vi "__package_structure.vi"(1 "data":string="Single shunt, R(Z1), 1kohm, S/N: 5\u0000\u0000                                                                                                                                                                                                                                                                                                                                                                                                                                                                                                                                                                                                                                                                                                                                                                                                                                                                                                                                                                                                    í\u0004\u0001\u0001\u0001\u0000\u0000\u0000\u0000\u0000\u0000?\u0007zD²ôç´\u0000\u0000?\u0007zD²ôgµ\u0000\u0000\u0000@\u0007zD²ôçµ\u0000\u0000@\u0007zD²ôg¶\u0000\u0000\u0000A\u0007zD²ôç¶\u0000\u0000A\u0007zD²ôg·\u0000\u0000\u0000B\u0007zD²ôç·\u0000\u0000B\u0007zD²ôg¸\u0000\u0000\u0000C\u0007zD²ôç¸\u0000\u0000C\u0007zD²ôg¹\u0000\u0000\u0000D\u0007zD²ôç¹\u0000\u0000D\u0007zD²ôgº\u0000\u0000\u0000E\u0007zD²ôçº\u0000\u0000E\u0007zD²ôg»\u0000\u0000\u0000F\u0007zD²ôç»\u0000\u0000F\u0007zD±ôg¼\u0000\u0000\u0000G\u0007zD±ôç¼\u0000\u0000G\u0007zD­ôg½\u0000\u0000\u0000H~\u0007zDôç½\u0000\u0000H\u001e\u0007zDcôg¾\u0000\u0000\u0000I\u0005zDuóç¾\u0011Mÿÿÿÿÿÿÿÿÿÿÿÿÿÿÿÿÿÿÿÿÿÿÿÿÿÿÿÿÿÿÿÿÿÿÿÿÿÿÿÿÿÿÿÿÿÿÿÿÿÿÿÿÿÿÿÿÿÿÿÿÿÿÿÿÿÿÿÿÿÿÿÿÿÿÿÿÿÿÿÿÿÿÿÿÿÿÿÿÿÿÿÿÿÿÿÿÿÿÿÿÿÿÿÿÿÿÿÿÿÿÿÿÿÿÿÿÿÿÿÿÿÿÿÿÿÿÿÿÿÿÿÿÿÿÿÿÿÿÿÿÿÿÿÿÿÿÿÿÿÿÿÿÿÿÿÿÿÿÿÿÿÿÿÿÿÿÿÿÿÿÿÿÿÿÿÿÿÿÿÿÿÿÿÿÿÿÿÿÿÿÿÿÿÿÿÿÿÿÿÿÿÿÿÿÿÿÿÿÿÿÿÿÿÿÿÿÿÿÿÿÿÿÿÿÿÿÿÿÿÿÿÿÿÿÿÿÿÿÿÿÿÿÿÿÿÿÿÿÿÿÿÿÿÿÿÿÿÿÿÿÿÿÿÿÿÿÿÿÿÿÿÿÿÿÿÿÿÿÿÿÿÿÿÿÿÿÿÿÿÿÿÿÿÿÿÿÿÿÿÿÿÿÿÿÿÿÿÿÿÿÿÿÿÿÿÿÿÿÿÿÿÿÿÿÿÿÿÿÿÿÿÿÿÿÿÿÿÿÿÿÿÿÿÿÿÿÿÿÿÿÿÿÿÿÿÿÿÿÿÿÿÿÿÿÿÿÿÿÿÿÿÿÿÿÿÿÿÿÿÿÿÿÿÿÿÿÿÿÿÿÿÿÿÿÿÿÿÿÿÿÿÿÿÿÿÿÿÿÿÿÿÿÿÿÿÿÿÿÿÿÿÿÿÿÿÿÿÿÿÿÿÿÿÿÿÿÿÿÿÿÿÿÿÿÿÿÿÿÿÿÿÿÿÿÿÿÿÿÿÿÿÿÿÿÿÿÿÿÿÿÿÿÿÿÿÿÿÿÿÿÿÿÿÿÿÿÿÿÿÿÿÿÿÿÿÿÿÿÿÿÿÿÿÿÿÿÿÿÿÿÿÿÿÿÿÿÿÿÿÿÿÿÿÿÿÿÿÿÿÿÿÿÿÿÿÿÿÿÿÿÿÿÿÿÿÿÿÿÿÿÿÿÿÿÿÿÿÿÿÿÿÿÿÿÿÿÿÿÿÿÿÿÿÿÿÿÿÿÿÿÿÿÿÿÿÿÿÿÿÿÿÿÿÿÿÿÿÿÿÿÿÿÿÿÿÿÿÿÿÿÿÿÿÿÿÿÿÿÿÿÿÿÿÿÿÿÿÿÿÿÿÿÿÿÿÿÿÿÿÿÿÿÿÿÿÿÿÿÿÿÿÿÿÿÿÿÿÿÿÿÿÿÿÿÿÿÿÿÿÿÿÿÿÿÿÿÿÿÿÿÿÿÿÿÿÿÿÿÿÿÿÿÿÿÿÿÿÿÿÿÿÿÿÿÿÿÿÿÿÿÿÿÿÿÿÿÿÿÿÿÿÿÿÿÿÿÿÿÿÿÿÿÿÿÿÿÿÿÿÿÿÿÿÿÿÿÿÿÿÿÿÿÿÿÿÿÿÿÿÿÿÿÿÿÿÿÿÿÿÿÿÿÿÿÿÿÿÿÿÿÿÿÿÿÿÿÿÿÿÿÿÿÿÿÿÿÿÿÿÿÿÿÿÿÿÿÿÿÿÿÿÿÿÿÿÿÿÿÿÿÿÿÿÿÿÿÿÿÿÿÿÿÿÿÿÿÿÿÿÿÿÿÿÿÿÿÿÿÿÿÿÿÿÿÿÿÿÿÿÿÿÿÿÿÿÿÿÿÿÿÿÿÿÿÿÿÿÿÿÿÿÿÿÿÿÿÿÿÿÿÿÿÿÿÿÿÿÿÿÿÿÿÿÿÿÿÿÿÿÿÿÿÿÿÿÿÿÿÿÿÿÿÿÿÿÿÿÿÿÿÿÿÿÿÿÿÿÿÿÿÿÿÿÿÿÿÿÿÿÿÿÿÿÿÿÿÿÿÿÿÿÿÿÿÿÿÿÿÿÿÿÿÿÿÿÿÿÿÿÿÿÿÿÿÿÿÿÿÿÿÿÿÿÿÿÿÿÿÿÿÿÿÿÿÿÿÿÿÿÿÿÿÿÿÿÿÿÿÿÿÿÿÿÿÿÿÿÿÿÿÿÿÿÿÿÿÿÿÿÿÿÿÿÿÿÿÿÿÿÿÿÿÿÿÿÿÿÿÿÿÿÿÿÿÿÿÿÿÿÿÿÿÿÿÿÿÿÿÿÿÿÿÿÿÿÿÿÿÿÿÿÿÿÿÿÿÿÿÿÿÿÿÿÿÿÿÿÿÿÿÿÿÿÿÿÿÿÿÿÿÿÿÿÿÿÿÿÿÿÿÿÿÿÿÿÿÿÿÿÿÿÿÿÿÿÿÿÿÿÿÿÿÿÿÿÿÿÿÿÿÿÿÿÿÿÿÿÿÿÿÿÿÿÿÿÿÿÿÿÿÿÿÿÿÿÿÿÿÿÿÿÿÿÿÿÿÿÿÿÿÿÿÿÿÿÿÿÿÿÿÿÿÿÿÿÿÿÿÿÿÿÿÿÿÿÿÿÿÿÿÿÿÿÿÿÿÿÿÿÿÿÿÿÿÿÿÿÿÿÿÿÿÿÿÿÿÿÿÿÿÿÿÿÿÿÿÿÿÿÿÿÿÿÿÿÿÿÿÿÿÿÿÿÿÿÿÿÿÿÿÿÿÿÿÿÿÿÿÿÿÿÿÿÿÿÿÿÿÿÿÿÿÿÿÿÿÿÿÿÿÿÿÿÿÿÿÿÿÿÿÿÿÿÿÿÿÿÿÿÿÿÿÿÿÿÿÿÿÿÿÿÿÿÿÿÿÿÿÿÿÿÿÿÿÿÿÿÿÿÿÿÿÿÿÿÿÿÿÿÿÿÿÿÿÿÿÿÿÿÿÿÿÿÿÿÿÿÿÿÿÿÿÿÿÿÿÿÿÿÿÿÿÿÿÿÿÿÿÿÿÿÿÿÿÿÿÿÿÿÿÿÿÿÿÿÿÿÿÿÿÿÿÿÿÿÿÿÿÿÿÿÿÿÿÿÿÿÿÿÿÿÿÿÿÿÿÿÿÿÿÿÿÿÿÿÿÿÿÿÿÿÿÿÿÿÿÿÿÿÿÿÿÿÿÿÿÿÿÿÿÿÿÿÿÿÿÿÿÿÿÿÿÿÿÿÿÿÿÿÿÿÿÿÿÿÿÿÿÿÿÿÿÿÿÿÿÿÿÿÿÿÿÿÿÿÿÿÿÿÿÿÿÿÿÿÿÿÿÿÿÿÿÿÿÿÿÿÿÿÿÿÿÿÿÿÿÿÿÿÿÿÿÿÿÿÿÿÿÿÿÿÿÿÿÿÿÿÿÿÿÿÿÿÿÿÿÿÿÿÿÿÿÿÿÿÿÿÿÿÿÿÿÿÿÿÿÿÿÿÿÿÿÿÿÿÿÿÿÿÿÿÿÿÿÿÿÿÿÿÿÿÿÿÿÿÿÿÿÿÿÿÿÿÿÿÿÿÿÿÿÿÿÿÿÿÿÿÿÿÿÿÿÿÿÿÿÿÿÿÿÿÿÿÿÿÿÿÿÿÿÿÿÿÿÿÿÿÿÿÿÿÿÿÿÿÿÿÿÿÿÿÿÿÿÿÿÿÿÿÿÿÿÿÿÿÿÿÿÿÿÿÿÿÿÿÿÿÿÿÿÿÿÿÿÿÿÿÿÿÿÿÿÿÿÿÿÿÿÿÿÿÿÿÿÿÿÿÿÿÿÿÿÿÿÿÿÿÿÿÿÿÿÿÿÿÿÿÿÿÿÿÿÿÿÿÿÿÿÿÿÿÿÿÿÿÿÿÿÿÿÿÿÿÿÿÿÿÿÿÿÿÿÿÿÿÿÿÿÿÿÿÿÿÿÿÿÿÿÿÿÿÿÿÿÿÿÿÿÿÿÿÿÿÿÿÿÿÿÿÿÿÿÿÿÿÿÿÿÿÿÿÿÿÿÿÿÿÿÿÿÿÿÿÿÿÿÿÿÿÿÿÿÿÿÿÿÿÿÿÿÿÿÿÿÿÿÿÿÿÿÿÿÿÿÿÿÿÿÿÿÿÿÿÿÿÿÿÿÿÿÿÿÿÿÿÿÿÿÿÿÿÿÿÿÿÿÿÿÿÿÿÿÿÿÿÿÿÿÿÿÿÿÿÿÿÿÿÿÿÿÿÿÿÿÿÿÿÿÿÿÿÿÿÿÿÿÿÿÿÿÿÿÿÿÿÿÿÿÿÿÿÿÿÿÿÿÿÿÿÿÿÿÿÿÿÿÿÿÿÿÿÿÿÿÿÿÿÿÿÿÿÿÿÿÿÿÿÿÿÿÿÿÿÿÿÿÿÿÿÿÿÿÿÿÿÿÿÿÿÿÿÿÿÿÿÿÿÿÿÿÿÿÿÿÿÿÿÿÿÿÿÿÿÿÿÿÿÿÿÿÿÿÿÿÿÿÿÿÿÿÿÿÿÿÿÿÿÿÿÿÿÿÿÿÿÿÿÿÿÿÿÿÿÿÿÿÿÿÿÿÿÿÿÿÿÿÿÿÿÿÿÿÿÿÿÿÿÿÿÿÿÿÿÿÿÿÿÿÿÿÿÿÿÿÿÿÿÿÿÿÿÿÿÿÿÿÿÿÿÿÿÿÿÿÿÿÿÿÿÿÿÿÿÿÿÿÿÿÿÿÿÿÿÿÿÿÿÿÿÿÿÿÿÿÿÿÿÿÿÿÿÿÿÿÿÿÿÿÿÿÿÿÿÿÿÿÿÿÿÿÿÿÿÿÿÿÿÿÿÿÿÿÿÿÿÿÿÿÿÿÿÿÿÿÿÿÿÿÿÿÿÿÿÿÿÿÿÿÿÿÿÿÿÿÿÿÿÿÿÿÿÿÿÿÿÿÿÿÿÿÿÿÿÿÿÿÿÿÿÿÿÿÿÿÿÿÿÿÿÿÿÿÿÿÿÿÿÿÿÿÿÿÿÿÿÿÿÿÿÿÿÿÿÿÿÿÿÿÿÿÿÿÿÿÿÿÿÿÿÿÿÿÿÿÿÿÿÿÿÿÿÿÿÿÿÿÿÿÿÿÿÿÿÿÿÿÿÿÿÿÿÿÿÿÿÿÿÿÿÿÿÿÿÿÿÿÿÿÿÿÿÿÿÿÿÿÿÿÿÿÿÿÿÿÿÿÿÿÿÿÿÿÿÿÿÿÿÿÿÿÿÿÿÿÿÿÿÿÿÿÿÿÿÿÿÿÿÿÿÿÿÿÿÿÿÿÿÿÿÿÿÿÿÿÿÿÿÿÿÿÿÿÿÿÿÿÿÿÿÿÿÿÿÿÿÿÿÿÿÿÿÿÿÿÿÿÿÿÿÿÿÿÿÿÿÿÿÿÿÿÿÿÿÿÿÿÿÿÿÿÿÿÿÿÿÿÿÿÿÿÿÿÿÿÿÿÿÿÿÿÿÿÿÿÿÿÿÿÿÿÿÿÿÿÿÿÿÿÿÿÿÿÿÿÿÿÿÿÿÿÿÿÿÿÿÿÿÿÿÿÿÿÿÿÿÿÿÿÿÿÿÿÿÿÿÿÿÿÿÿÿÿÿÿÿÿÿÿÿÿÿÿÿÿÿÿÿÿÿÿÿÿÿÿÿÿÿÿÿÿÿÿÿÿÿÿÿÿÿÿÿÿÿÿÿÿÿÿÿÿÿÿÿÿÿÿÿÿÿÿÿÿÿÿÿÿÿÿÿÿÿÿÿÿÿÿÿÿÿÿÿÿÿÿÿÿÿÿÿÿÿÿÿÿÿÿÿÿÿÿÿÿÿÿÿÿÿÿÿÿÿÿÿÿÿÿÿÿÿÿÿÿÿÿÿÿÿÿÿÿÿÿÿÿÿÿÿÿÿÿÿÿÿÿÿÿÿÿÿÿÿÿÿÿÿÿÿÿÿÿÿÿÿÿÿÿÿÿÿÿÿÿÿÿÿÿÿÿÿÿÿÿÿÿÿÿÿÿÿÿÿÿÿÿÿÿÿÿÿÿÿÿÿÿÿÿÿÿÿÿÿÿÿÿÿÿ\u0001\u0000\u0003\u0000\u0000\u0000\u0000ÿÿÿÿÿÿÿÿÿÿÿÿÿÿÿÿÿÿÿÿÿÿÿÿÿÿÿÿÿÿÿÿÿÿÿÿÿÿÿÿÿÿÿÿÿÿÿÿÿÿÿÿÿÿÿÿÿÿÿÿÿÿÿÿÿÿÿÿÿÿÿÿÿÿÿÿÿÿÿÿÿÿÿÿÿÿÿÿÿÿÿÿÿÿÿÿÿÿÿÿÿÿÿÿÿÿÿÿÿÿÿÿÿÿÿÿÿÿÿÿÿÿÿÿÿÿÿÿÿÿÿÿÿÿÿÿÿÿÿÿÿÿÿÿÿÿÿÿÿÿÿÿÿÿÿÿÿÿÿÿÿÿÿÿÿÿÿÿÿÿÿÿÿÿÿÿÿÿÿÿÿÿÿÿÿÿÿÿÿÿÿÿÿÿÿÿÿÿÿÿÿÿÿÿÿÿÿÿÿÿÿÿÿÿÿÿÿÿÿÿÿÿÿÿÿÿÿÿÿÿÿÿÿÿÿÿÿÿÿÿÿÿÿÿÿÿÿÿÿÿÿÿÿÿÿÿÿÿÿÿÿÿÿÿÿÿÿÿÿÿÿÿÿÿÿÿÿÿÿÿÿÿÿÿÿÿÿÿÿÿÿÿÿÿÿÿÿÿÿÿÿÿÿÿÿÿÿÿÿÿÿÿÿÿÿÿÿÿÿÿÿÿÿÿÿÿÿÿÿÿÿÿÿÿÿÿÿÿÿÿÿÿÿÿÿÿÿÿÿÿÿÿÿÿÿÿÿÿÿÿÿÿÿÿÿÿÿÿÿÿÿÿÿÿÿÿÿÿÿÿÿÿÿÿÿÿÿÿÿÿÿÿÿÿÿÿÿÿÿÿÿÿÿÿÿÿÿÿÿÿÿÿÿÿÿÿÿÿÿÿÿÿÿÿÿÿÿÿÿÿÿÿÿÿÿÿÿÿÿÿÿÿÿÿÿÿÿÿÿÿÿÿÿÿÿÿÿÿÿÿÿÿÿÿÿÿÿÿÿÿÿÿÿÿÿÿÿÿÿÿÿÿÿÿÿÿÿÿÿÿÿÿÿÿÿÿÿÿÿÿÿÿÿÿÿÿÿÿÿÿÿÿÿÿÿÿÿÿÿÿÿÿÿÿÿÿÿÿÿÿÿÿÿÿÿÿÿÿÿÿÿÿÿÿÿÿÿÿÿÿÿÿÿÿÿÿÿÿÿÿÿÿÿÿÿÿÿÿÿÿÿÿÿÿÿÿÿÿÿÿÿÿÿÿÿÿÿÿÿÿÿÿÿÿÿÿÿÿÿÿÿÿÿÿÿÿÿÿÿÿÿÿÿÿÿÿÿÿÿÿÿÿÿÿÿÿÿÿÿÿÿÿÿÿÿÿÿÿÿÿÿÿÿÿÿÿÿÿÿÿÿÿÿÿÿÿÿÿÿÿÿÿÿÿÿÿÿÿÿÿÿÿÿÿÿÿÿÿÿÿÿÿÿÿÿÿÿÿÿÿÿÿÿÿÿÿÿÿÿÿÿÿÿÿÿÿÿÿÿÿÿÿÿÿÿÿÿÿÿÿÿÿÿÿÿÿÿÿÿÿÿÿÿÿÿÿÿÿÿÿÿÿÿÿÿÿÿÿÿÿÿÿÿÿÿÿÿÿÿÿÿÿÿÿÿÿÿÿÿÿÿÿÿÿÿÿÿÿÿÿÿÿÿÿÿÿÿÿÿÿÿÿÿÿÿÿÿÿÿÿÿÿÿÿÿÿÿÿÿÿÿÿÿÿÿÿÿÿÿÿÿÿÿÿÿÿÿÿÿÿÿÿÿÿÿÿÿÿÿÿÿÿÿÿÿÿÿÿÿÿÿÿÿÿÿÿÿÿÿÿÿÿÿÿÿÿÿÿÿÿÿÿÿÿÿÿÿÿÿÿÿÿÿÿÿÿÿÿÿÿÿÿÿÿÿÿÿÿÿÿÿÿÿÿÿÿÿÿÿÿÿÿÿÿÿÿÿÿÿÿÿÿÿÿÿÿÿÿÿÿÿÿÿÿÿÿÿÿÿÿÿÿÿÿÿÿÿÿÿÿÿÿÿÿÿÿÿÿÿÿÿÿÿÿÿÿÿÿÿÿÿÿÿÿÿÿÿÿÿÿÿÿÿÿÿÿÿÿÿÿÿÿÿÿÿÿÿÿÿÿÿÿÿÿÿÿÿÿÿÿÿÿÿÿÿÿÿÿÿÿÿÿÿÿÿÿÿÿÿÿÿÿÿÿÿÿÿÿÿÿÿÿÿÿÿÿÿÿÿÿÿÿÿÿÿÿÿÿÿÿÿÿÿÿÿÿÿÿÿÿÿÿÿÿÿÿÿÿÿÿÿÿÿÿÿÿÿÿÿÿÿÿÿÿÿÿÿÿÿÿÿÿÿÿÿÿÿÿÿÿÿÿÿÿÿÿÿÿÿÿÿÿÿÿÿÿÿÿÿÿÿÿÿÿÿÿÿÿÿÿÿÿÿÿÿÿÿÿÿÿÿÿÿÿÿÿÿÿÿÿÿÿÿÿÿÿÿÿÿÿÿÿÿÿÿÿÿÿÿÿÿÿÿÿÿÿÿÿÿÿÿÿÿÿÿÿÿÿÿÿÿÿÿÿÿÿÿÿÿÿÿÿÿÿÿÿÿÿÿÿÿÿÿÿÿÿÿÿÿÿÿÿÿÿÿÿÿÿÿÿÿÿÿÿÿÿÿÿÿÿÿÿÿÿÿÿÿÿÿÿÿÿÿÿÿÿÿÿÿÿÿÿÿÿÿÿÿÿÿÿÿÿÿÿÿÿÿÿÿÿÿÿÿÿÿÿÿÿÿÿÿÿÿÿÿÿÿÿÿÿÿÿÿÿÿÿÿÿÿÿÿÿÿÿÿÿÿÿÿÿÿÿÿÿÿÿÿÿÿÿÿÿÿÿÿÿÿÿÿÿÿÿÿÿÿÿÿÿÿÿÿÿÿÿÿÿÿÿÿÿÿÿÿÿÿÿÿÿÿÿÿÿÿÿÿÿÿÿÿÿÿÿÿÿÿÿÿÿÿÿÿÿÿÿÿÿÿÿÿÿÿÿÿÿÿÿÿÿÿÿÿÿÿÿÿÿÿÿÿÿÿÿÿÿÿÿÿÿÿÿÿÿÿÿÿÿÿÿÿÿÿÿÿÿÿÿÿÿÿÿÿÿÿÿÿÿÿÿÿÿÿÿÿÿÿÿÿÿÿÿÿÿÿÿÿÿÿÿÿÿÿÿÿÿÿÿÿÿÿÿÿÿÿÿÿÿÿÿÿÿÿÿÿÿÿÿÿÿÿÿÿÿÿÿÿÿÿÿÿÿÿÿÿÿÿÿÿÿÿÿÿÿÿÿÿÿÿÿÿÿÿÿÿÿÿÿÿÿÿÿÿÿÿÿÿÿÿÿÿÿÿÿÿÿÿÿÿÿÿÿÿÿÿÿÿÿÿÿÿÿÿÿÿÿÿÿÿÿÿÿÿÿÿÿÿÿÿÿÿÿÿÿÿÿÿÿÿÿÿÿÿÿÿÿÿÿÿÿÿÿÿÿÿÿÿÿÿÿÿÿÿÿÿÿÿÿÿÿÿÿÿÿÿÿÿÿÿÿÿÿÿÿÿÿÿÿÿÿÿÿÿÿÿÿÿÿÿÿÿÿÿÿÿÿÿÿÿÿÿÿÿÿÿÿÿÿÿÿÿÿÿÿÿÿÿÿÿÿÿÿÿÿÿÿÿÿÿÿÿÿÿÿÿÿÿÿÿÿÿÿÿÿÿÿÿÿÿÿÿÿÿÿÿÿÿÿÿÿÿÿÿÿÿÿÿÿÿÿÿÿÿÿÿÿÿÿÿÿÿÿÿÿÿÿÿÿÿÿÿÿÿÿÿÿÿÿÿÿÿÿÿÿÿÿÿÿÿÿÿÿÿÿÿÿÿÿÿÿÿÿÿÿÿÿÿÿÿÿÿÿÿÿÿÿÿÿÿÿÿÿÿÿÿÿÿÿÿÿÿÿÿÿÿÿÿÿÿÿÿÿÿÿÿÿÿÿÿÿÿÿÿÿÿÿÿÿÿÿÿÿÿÿÿÿÿÿÿÿÿÿÿÿÿÿÿÿÿÿÿÿÿÿÿÿÿÿÿÿÿÿÿÿÿÿÿÿÿÿÿÿÿÿÿÿÿÿÿÿÿÿÿÿÿÿÿÿÿÿÿÿÿÿÿÿÿÿÿÿÿÿÿÿÿÿÿÿÿÿÿÿÿÿÿÿÿÿÿÿÿÿÿÿÿÿÿÿÿÿÿÿÿÿÿÿÿÿÿÿÿÿÿÿÿÿÿÿÿÿÿÿÿÿÿÿÿÿÿÿÿÿÿÿÿÿÿÿÿÿÿÿÿÿÿÿÿÿÿÿÿÿÿÿÿÿÿÿÿÿÿÿÿÿÿÿÿÿÿÿÿÿÿÿÿÿÿÿÿÿÿÿÿÿÿÿÿÿÿÿÿÿÿÿÿÿÿÿÿÿÿÿÿÿÿÿÿÿÿÿÿÿÿÿÿÿÿÿÿÿÿÿÿÿÿÿÿÿÿÿÿÿÿÿÿÿÿÿÿÿÿÿÿÿÿÿÿÿÿÿÿÿÿÿÿÿÿÿÿÿÿÿÿÿÿÿÿÿÿÿÿÿÿÿÿÿÿÿÿÿÿÿÿÿÿÿÿÿÿÿÿÿÿÿÿÿÿÿÿÿÿÿÿÿÿÿÿÿÿÿÿÿÿÿÿÿÿÿÿÿÿÿÿÿÿÿÿÿÿÿÿÿÿÿÿÿÿÿÿÿÿÿÿÿÿÿÿÿÿÿÿÿÿÿÿÿÿÿÿÿÿÿÿÿÿÿÿÿÿÿÿÿÿÿÿÿÿÿÿÿÿÿÿÿÿÿÿÿÿÿÿÿÿÿÿÿÿÿÿÿÿÿÿÿÿÿÿÿÿÿÿÿÿÿÿÿÿÿÿÿÿÿÿÿÿÿÿÿÿÿÿÿÿÿÿÿÿÿÿÿÿÿÿÿÿÿÿÿÿÿÿÿÿÿÿÿÿÿÿÿÿÿÿÿÿÿÿÿÿÿÿÿÿÿÿÿÿÿÿÿÿÿÿÿÿÿÿÿÿÿÿÿÿÿÿÿÿÿÿÿÿÿÿÿÿÿÿÿÿÿÿÿÿÿÿÿÿÿÿÿÿÿÿÿÿÿÿÿÿÿÿÿÿÿÿÿÿÿÿÿÿÿÿÿÿÿÿÿÿÿÿÿÿÿÿÿÿÿÿÿÿÿÿÿÿÿÿÿÿÿÿÿÿÿÿÿÿÿÿÿÿÿÿÿÿÿÿÿÿÿÿÿÿÿÿÿÿÿÿÿÿÿÿÿÿÿÿÿÿÿÿÿÿÿÿÿÿÿÿÿÿÿÿÿÿÿÿÿÿÿÿÿÿÿÿÿÿÿÿÿÿÿÿÿÿÿÿÿÿÿÿÿÿÿÿÿÿÿÿÿÿÿÿÿÿÿÿÿÿÿÿÿÿÿÿÿÿÿÿÿÿÿÿÿÿÿÿÿÿÿÿÿÿÿÿÿÿÿÿÿÿÿÿÿÿÿÿÿÿÿÿÿÿÿÿÿÿÿÿÿÿÿÿÿÿÿÿÿÿÿÿÿÿÿÿÿÿÿÿÿÿÿÿÿÿÿÿÿÿÿÿÿÿÿÿÿÿÿÿÿÿÿÿÿÿÿÿÿÿÿÿÿÿÿÿÿÿÿÿÿÿÿÿÿÿÿÿÿÿÿÿÿÿÿÿÿÿÿÿÿÿÿÿÿÿÿÿÿÿÿÿÿÿÿÿÿÿÿÿÿÿÿÿÿÿÿÿÿÿÿÿÿÿÿÿÿÿÿÿÿÿÿÿÿÿÿÿÿÿÿÿÿÿÿÿÿÿÿÿÿÿÿÿÿÿÿÿÿÿÿÿÿÿÿÿÿÿÿÿÿÿÿÿÿÿÿÿÿÿÿÿÿÿÿÿÿÿÿÿÿÿÿÿÿÿÿÿÿÿÿÿÿÿÿÿÿÿÿÿÿÿÿÿÿÿÿÿÿÿÿÿÿÿÿÿÿÿÿÿÿÿÿÿÿÿÿÿÿÿÿÿÿÿÿÿÿÿÿÿÿÿÿÿÿÿÿÿÿÿÿÿÿÿÿÿÿÿÿÿÿÿÿÿÿÿÿÿÿÿÿÿÿÿÿÿÿÿÿÿÿÿÿÿÿÿÿÿÿÿÿÿÿÿÿÿÿÿÿÿÿÿÿÿÿÿÿÿÿÿÿÿÿÿÿÿÿÿÿÿÿÿÿÿÿÿÿÿÿÿÿÿÿÿÿÿÿÿÿÿÿÿÿÿÿÿÿÿÿÿÿÿÿÿÿÿÿÿÿÿÿÿÿÿÿÿÿÿÿÿÿÿÿÿÿÿÿÿÿÿÿÿÿÿÿÿÿÿÿÿÿÿÿÿÿÿÿÿÿÿÿÿÿÿÿÿÿÿÿÿÿÿÿÿÿÿÿÿÿÿÿÿÿÿÿÿÿÿÿÿÿÿÿÿÿÿÿÿÿÿÿÿÿÿÿÿÿÿÿÿÿÿÿÿÿÿÿÿÿÿÿÿÿÿÿÿÿÿÿÿÿÿÿÿÿÿÿÿÿÿÿÿÿÿÿÿÿÿÿÿÿÿÿÿÿÿÿÿÿÿÿÿÿÿÿÿÿÿÿÿÿÿÿÿÿÿÿÿÿÿÿÿÿÿÿÿÿÿÿÿÿÿÿÿÿÿÿÿÿÿÿÿÿÿÿÿÿÿÿÿÿÿÿÿÿÿÿÿÿÿÿÿÿÿÿÿÿÿÿÿÿÿÿÿÿÿÿÿÿÿÿÿÿÿÿÿÿÿÿÿÿÿÿÿÿÿÿÿÿÿÿÿÿÿÿÿÿÿÿÿÿÿÿÿÿÿÿÿÿÿÿÿÿÿÿÿÿÿÿÿÿÿÿÿÿÿÿÿÿÿÿÿÿÿÿÿÿÿÿÿÿÿÿÿÿÿÿÿÿÿÿÿÿÿÿÿÿÿÿÿÿÿÿÿÿÿÿÿÿÿÿÿÿÿÿÿÿÿÿÿÿÿÿÿÿÿÿÿÿÿÿÿÿÿÿÿÿÿÿÿÿÿÿÿÿÿÿÿÿÿÿÿÿÿÿÿÿÿÿÿÿÿÿÿÿÿÿÿÿÿÿÿÿÿÿÿÿÿÿÿÿÿÿÿÿÿÿÿÿÿÿÿÿÿÿÿÿÿÿÿÿÿÿÿÿÿÿÿÿÿÿÿÿÿÿÿÿÿÿÿÿÿÿÿÿÿÿÿÿÿÿÿÿÿÿÿÿÿÿÿÿÿÿÿÿÿÿÿÿÿÿÿÿÿÿÿÿÿÿÿÿÿÿÿÿÿÿÿÿÿÿÿÿÿÿÿÿÿÿÿÿÿÿÿÿÿÿÿÿÿÿÿÿÿÿÿÿÿÿÿÿÿÿÿÿÿÿÿÿÿÿÿÿÿÿÿÿÿÿÿÿÿÿÿÿÿÿÿÿÿÿÿÿÿÿÿÿÿÿÿÿÿÿÿÿÿÿÿÿÿÿÿÿÿÿÿÿÿÿÿÿÿÿÿÿÿÿÿÿÿÿÿÿÿÿÿÿÿÿÿÿÿÿÿÿÿÿÿÿÿÿÿÿÿÿÿÿÿÿÿÿÿÿÿÿÿÿÿÿÿÿÿÿÿÿÿÿÿÿÿÿÿÿÿÿÿÿÿÿÿÿÿÿÿÿÿÿÿÿÿÿÿÿÿÿÿÿÿÿÿÿÿÿÿÿÿÿÿÿÿÿÿÿÿÿÿÿÿÿÿÿÿÿÿÿÿÿÿÿÿÿÿÿÿÿÿÿÿÿÿÿÿÿÿÿÿÿÿÿÿÿÿÿÿÿÿÿÿÿÿÿÿÿÿÿÿÿÿÿÿÿÿÿÿÿÿÿÿÿÿÿÿÿÿÿÿÿÿÿÿÿÿÿÿÿÿÿÿÿÿÿÿÿÿÿÿÿÿÿÿÿÿÿÿÿÿÿÿÿÿÿÿÿÿÿÿÿÿÿÿÿÿÿÿÿÿÿÿÿÿÿÿÿÿÿÿÿÿÿÿÿÿÿÿÿÿÿÿÿÿÿÿÿÿÿÿÿÿÿÿÿÿÿÿÿÿÿÿÿÿÿÿÿÿÿÿÿÿÿÿÿÿÿÿÿÿÿÿÿÿÿÿÿÿÿÿÿÿ") -> (6 "size_status":u16[](array[numeric])=[192, 17, 192, 17, 192, 17, 192, 17, 192, 17, 192, 17, 192, 17, 192, 17, 192, 17, 192, 17, 192, 17, 192, 17, 192, 17, 192, 17, 192, 17, 192, 17, 192, 17, 192, 17, 192, 17, 192, 17, 192, 17, 192, 17, 192, 17, 192, 17, 192, 17, 192, 17, 192, 17, 192, 17, 192, 17, 192, 17], 7 "cycles":i32=30, 8 "count":u32[](array[numeric])=[179491, 179492, 179493, 179497, 179498, 179502, 179506, 179507, 179511, 179512, 179516, 179517], 10 "cycle period":u32[](array[numeric])=[990, 990, 986, 982, 989, 984, 987, 986, 993, 981, 992, 988, 983, 986, 990, 988, 986, 984, 988, 985, 989, 986, 989, 986, 986, 990, 989, 980, 991, 984], 11 "reserved":u16[](array[numeric]), 13 "to logfile":string[](array[string]), 15 "max_min":u16[](array[numeric])=[2123, 1935, 3621, 463, 2128, 1942, 3620, 464, 2130, 1945, 3621, 462, 1935, 1749, 3693, 408, 1943, 1759, 3692, 403, 2014, 1827, 3703, 398, 2277, 2055, 3450, 635, 2277, 2056, 3451, 635, 2137, 1952, 3618, 460, 2136, 1952, 3619, 461, 2019, 1835, 3693, 403, 2024, 1841, 3695, 402], 16 "M":sgl[][](array[numeric])=[[88.106, 83.85775, 48.398014, 59.123047, 55.20648, 54.99554, 56.17912, 55.418804, 56.6034, 55.430943, 55.49297, 56.396164, 56.69431, 57.245438, 58.198605], [68.15673, 70.64137, 53.270576, 57.542862, 55.985424, 55.310055, 56.012516, 55.89808, 56.228584, 55.327404, 55.385227, 56.345207, 56.69351, 57.18125, 58.154873], [61.696934, 65.15628, 54.834675, 56.314125, 56.25808, 55.7536, 55.8175, 55.87484, 56.207226, 55.398163, 55.611202, 56.23936, 56.742786, 57.367477, 58.112923], [108.64962, 79.99922, 45.719025, 56.21946, 51.952293, 51.368572, 52.483074, 51.638813, 52.811127, 51.658546, 51.7936, 52.431408, 52.950626, 53.74078, 54.61418], [83.89287, 71.57887, 47.63007, 55.203976, 52.56592, 51.55626, 52.070206, 51.721554, 52.654507, 51.622147, 51.786396, 52.488674, 53.06406, 53.766438, 54.521873], [62.136074, 51.99304, 54.359753, 52.178143, 53.90879, 53.122314, 52.900307, 53.385944, 53.6065, 52.955986, 53.250786, 53.961914, 54.461372, 55.221905, 56.153473], [76.99525, 83.32456, 75.389336, 76.76034, 76.65508, 76.399506, 76.18332, 76.10905, 76.62135, 75.92104, 75.89582, 76.37503, 76.9038, 77.18269, 77.4808], [77.42664, 81.41321, 75.64364, 76.8206, 76.156235, 75.73216, 76.24693, 76.18514, 76.84914, 75.85005, 75.71804, 76.4735, 76.834305, 77.148506, 77.6828], [62.482994, 57.840115, 57.08614, 55.503063, 56.433216, 55.59795, 55.61169, 55.952553, 56.38317, 55.270702, 55.631203, 56.148037, 56.65967, 57.269684, 57.990593], [60.486343, 60.011143, 56.83409, 56.083416, 56.254593, 55.64892, 55.95295, 56.090588, 56.5381, 55.33873, 55.593773, 56.223675, 56.742783, 57.31412, 58.26447], [81.46664, 73.40286, 46.214756, 54.75707, 52.241432, 51.770203, 52.255, 51.97851, 52.61516, 51.637928, 51.78695, 52.671387, 53.08716, 53.747433, 54.61967], [68.07129, 64.914955, 49.057117, 53.551888, 52.729916, 51.907322, 52.15726, 52.10843, 52.607555, 51.7876, 51.750725, 52.541878, 52.927555, 53.83889, 54.555595]], 17 "Ph":sgl[][](array[numeric])=[[67.755806, -5.316972, 13.839581, 1.9545214, 1.2133443, -1.3619734, -0.6751799, -0.50703865, 0.18179742, 0.35251305, 0.59943706, 1.181565, 1.496611, 1.5759457, 1.529413], [39.5804, -1.8039719, 6.3453693, 1.712283, 0.31226763, -0.6932076, -0.13438612, -0.2951022, -0.035128176, 0.22534728, 0.6655266, 1.1402423, 1.4711579, 1.6442983, 1.4962261], [30.254652, 0.010333736, 3.5842934, 1.2630581, -0.2641627, -0.5503447, -0.4353858, -0.533313, 0.008992521, 0.23606402, 0.57926315, 1.0986413, 1.3385687, 1.5040715, 1.421692], [67.71805, -8.868363, 18.208672, 1.8901482, 1.730241, -1.4529985, -0.63252145, -0.098414704, 0.48198688, 0.27106896, 0.81647784, 1.5975958, 1.4863187, 1.787064, 1.5321264], [54.447006, -6.562586, 11.472527, 1.2149398, 0.83358943, -1.3376569, -0.37363434, -0.23254518, 0.3666669, 0.4767456, 0.8522804, 1.553027, 1.5662773, 1.8375467, 1.4985178], [-7.5674286, 6.3610725, -0.9412131, 0.3655917, -0.6878183, 0.025334053, -0.09531969, -0.099220306, 0.4311631, 0.7247993, 1.010056, 1.5445243, 1.7237602, 1.890241, 1.6444137], [14.133752, 2.4586954, 2.8025115, 1.0280558, -0.22411773, -0.15571654, -0.1365338, -0.05708496, -0.06202886, 0.25595987, 0.15296178, 0.44356167, 0.7310988, 0.9726959, 0.91783184], [12.69936, 2.5250893, 2.6215646, 0.74278843, -0.09992821, 0.046831895, -0.22724898, 0.14888294, -0.03955752, 0.15902488, 0.16409843, 0.39973316, 0.5533274, 0.85644376, 0.9311564], [2.1667078, 5.6543126, 0.38095114, 0.5809965, -0.6891161, -0.23623835, -0.014240538, -0.28871146, -0.14875747, 0.30969292, 0.58636254, 1.1004258, 1.3726633, 1.5663401, 1.5098989], [6.969983, 3.8036287, 1.2874038, 0.62625283, -0.38749772, -0.3763116, -0.49575487, -0.4646439, -0.07050607, 0.51253676, 0.5976072, 1.2017618, 1.2586643, 1.6391829, 1.4776497], [59.189724, -5.2501, 12.6670265, 1.9459636, 0.831382, -1.2912755, -0.5476761, -0.32437295, 0.4842284, 0.35907775, 0.8273565, 1.3775605, 1.4734876, 1.7201649, 1.554983], [39.781384, -1.7384396, 6.7731733, 1.9458405, 0.059315365, -0.75686634, -0.43746033, -0.033024494, 0.47244552, 0.4212529, 1.0115715, 1.4187251, 1.5314804, 1.7837197, 1.5999893]], 18 "status":u16[](array[numeric])=[4299, 0, 6, 4299, 0, 6, 4299, 0, 6, 4299, 0, 7, 4299, 0, 7, 4299, 0, 6, 4299, 0, 5, 4299, 0, 5, 4299, 0, 4, 4299, 0, 4, 4299, 0, 5, 4299, 0, 5], 19 "to_logfile":sgl[][](array[numeric]))   [LabVIEW 2017, in "ZBOX_IS.lvlib"]
uses:
  ZBOX_IS.lvlib
panel:
  out "bytes":i32=5760
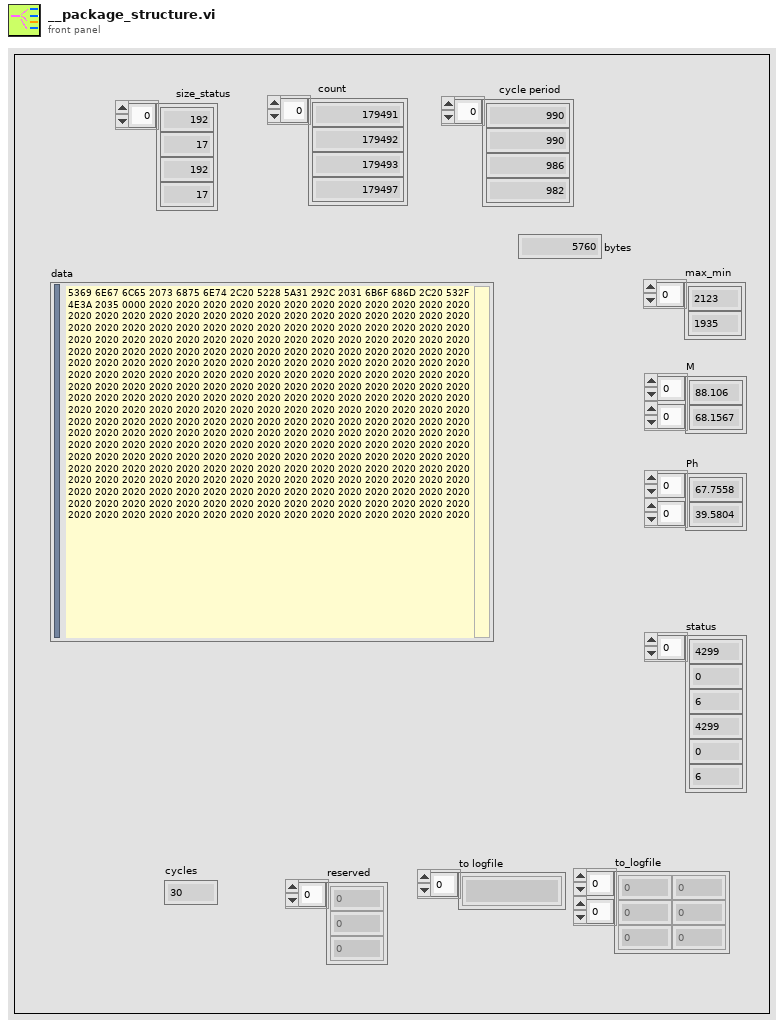
[diagram p1: front panel]
types:
  T1 = enum16{"big-endian, network order", "native, host order", "little-endian"}
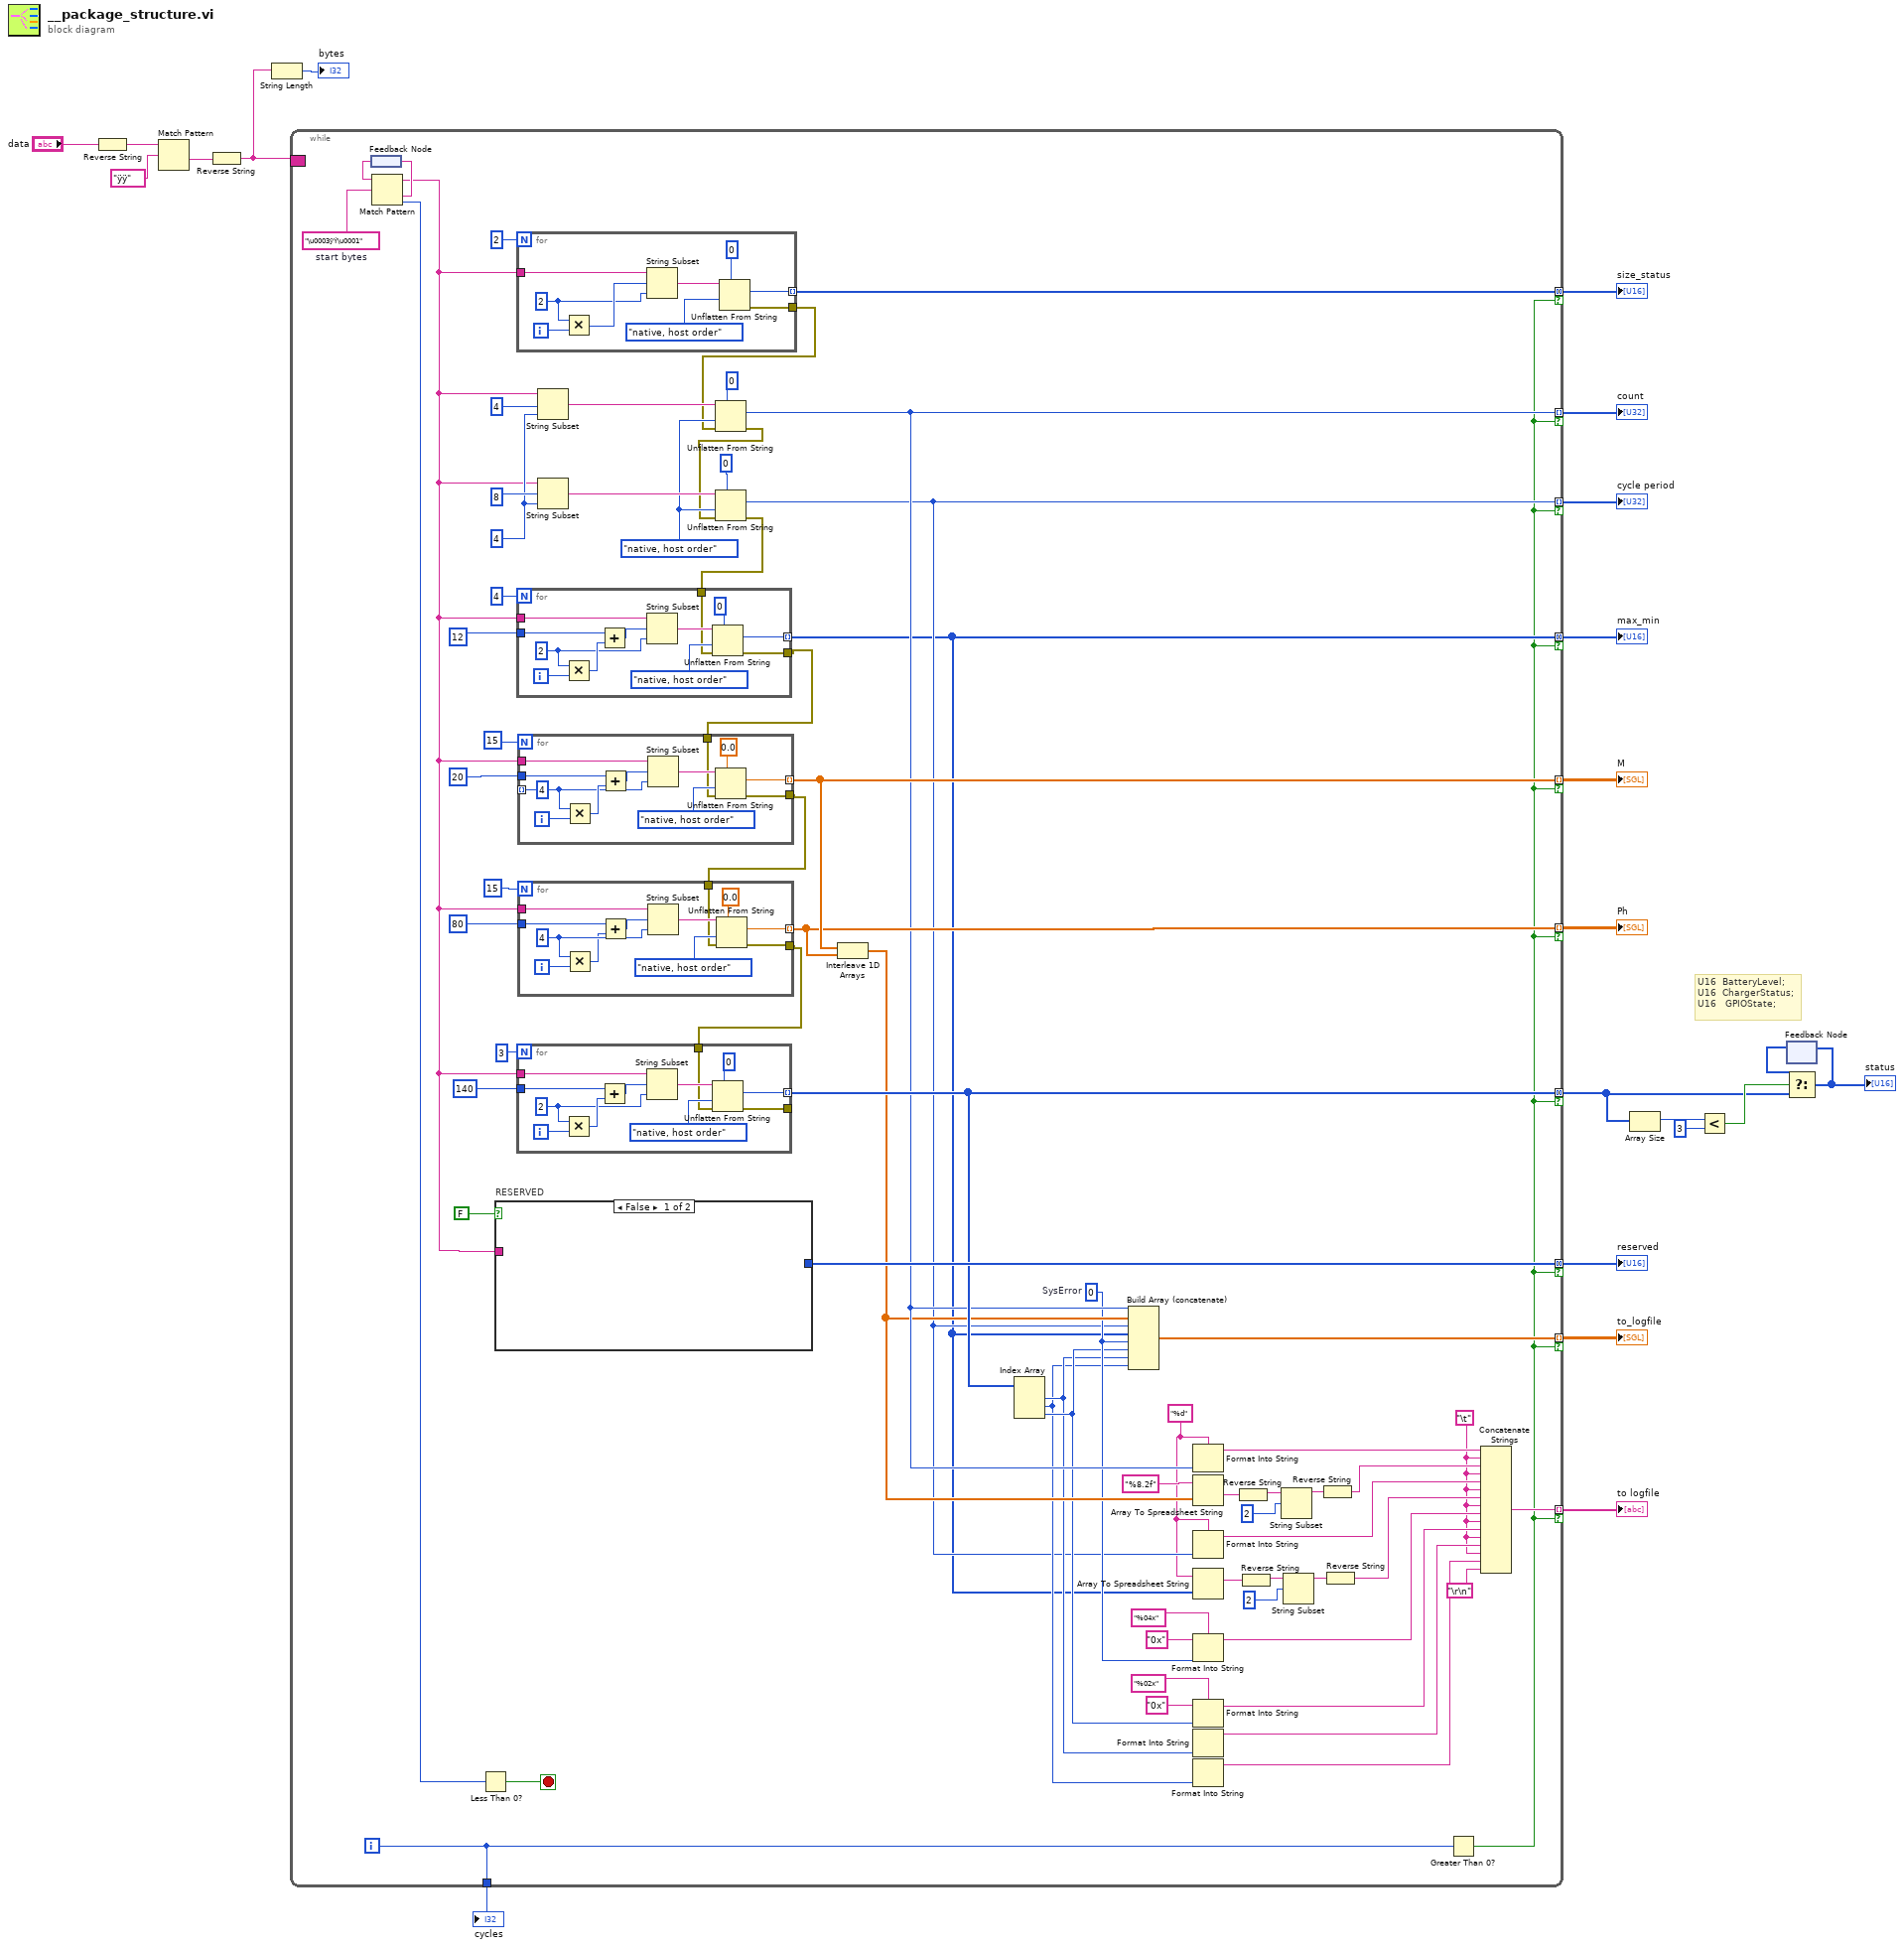
[diagram p0: block diagram]
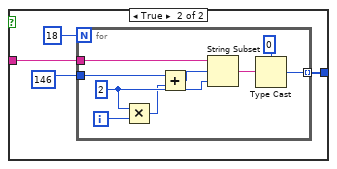
[diagram p2: hidden frame]
diagram:
  # "U16  BatteryLevel;\nU16  ChargerStatus;\nU16   GPIOState;"
  n1 = Reverse String(1:"data") -> (0:w7:string)
  n2 = Match Pattern(string=w7, regular expression="ÿÿ") -> (after substring=w5:string)  [unwired: 1 in, 3 out]
  n3 = Reverse String(1:w5) -> (0:w3:string)
  n4 = String Length(string=w3) -> (length=→"bytes":i32)
  n5 = while {
    border: w3 -> [_]
    tunnel: [w65] -> w16 mode=indexing if=w32
    tunnel: [w31] -> w20
    tunnel: [w47] -> w21 mode=concatenating if=w32
    tunnel: [w90] -> w22 mode=concatenating if=w32
    tunnel: [w89] -> w19 mode=concatenating if=w32
    tunnel: [w48] -> w18 mode=indexing if=w32
    tunnel: [w69] -> w15 mode=indexing if=w32
    tunnel: [w68] -> w17 mode=indexing if=w32
    tunnel: [w67] -> w2 mode=concatenating if=w32
    tunnel: [w66] -> w14 mode=indexing if=w32
    tunnel: [w49] -> w13 mode=indexing if=w32
    i -> [w31]
    stop <- w82 stop-if-true
    w23 = "\u0003ÿÝ\u0001"  # start bytes
    w46 = "%d" ("format string")
    w33 = "\t"
    w60 = 0  # SysError
    w83 = T1."native, host order" ("byte order (0:big-endian, network order) 2")
    w77 = 4 ("length (rest)")
    n6 = feedback #1() -> (w92:string)
    n7 = Match Pattern(string=w92, regular expression=w23) -> (before substring=w73:string, after substring=w93:string, offset past match=w86:i32)  [unwired: 1 in, 1 out]
    n8 = feedback-in #1(w93) -> ()
    n9 = Less Than 0?(x=w86) -> (x < 0?=w82:bool)
    n10 = case "RESERVED" shown="False" FALSE {
      tunnel: [_ w109] -> w90
      tunnel: w73 -> [_ w108]
      frame False {
      }
      frame True {
        n11 = for {
          N: 18 -> [_]
          tunnel: w108 -> [w118]
          tunnel: [w115] -> w109 mode=indexing
          tunnel: 146 ("Numeric") -> [w111]
          i -> [w114]
          w112 = 2 ("length (rest)")
          n12 = Multiply(x=w112, y=w114) -> (x*y=w110:i32)
          n13 = Add(x=w111, y=w110) -> (x+y=w113:i32)
          n14 = String Subset(string=w118, offset (0)=w113, length (rest)=w112) -> (substring=w117:string)
          n15 = Type Cast(type=u16 0, x=w117) -> (*(type *) &x=w115:u16)
        }
      }
    }
    n16 = for {
      N: 2 -> [_]
      tunnel: w73 -> [w139]
      tunnel: [w133] -> w89 mode=indexing
      tunnel: [w132] -> w29
      i -> [w138]
      w131 = 2 ("length (rest)")
      n17 = Multiply(x=w131, y=w138) -> (x*y=w137:i32)
      n18 = String Subset(string=w139, offset (0)=w137, length (rest)=w131) -> (substring=w136:string)
      n19 = Unflatten From String(type=u16 0, binary string=w136, byte order (0:big-endian, network order)=T1."native, host order" ("byte order (0:big-endian, network order) 2")) -> (value=w133:u16, error out=w132:errorcluster)  [unwired: 2 in, 1 out]
    }
    n20 = String Subset(string=w73, offset (0)=4, length (rest)=w77) -> (substring=w87:string)
    n21 = String Subset(string=w73, offset (0)=8, length (rest)=w77) -> (substring=w85:string)
    n22 = Unflatten From String(type=u32 0, binary string=w87, byte order (0:big-endian, network order)=w83, error in (no error)=w29) -> (value=w65:u32, error out=w28:errorcluster)  [unwired: 1 in, 1 out]
    n23 = Unflatten From String(type=u32 0, binary string=w85, byte order (0:big-endian, network order)=w83, error in (no error)=w28) -> (value=w48:u32, error out=w27:errorcluster)  [unwired: 1 in, 1 out]
    n24 = for {
      N: 4 -> [_]
      tunnel: w73 -> [w159]
      tunnel: [w158] -> w47 mode=indexing
      tunnel: 12 ("offset (0)") -> [w161]
      tunnel: [w157] -> w26
      tunnel: w27 -> [w152]
      i -> [w163]
      w153 = 2 ("length (rest)")
      n25 = Multiply(x=w153, y=w163) -> (x*y=w160:i32)
      n26 = Add(x=w161, y=w160) -> (x+y=w162:i32)
      n27 = String Subset(string=w159, offset (0)=w162, length (rest)=w153) -> (substring=w155:string)
      n28 = Unflatten From String(type=u16 0, binary string=w155, byte order (0:big-endian, network order)=T1."native, host order" ("byte order (0:big-endian, network order) 2"), error in (no error)=w152) -> (value=w158:u16, error out=w157:errorcluster)  [unwired: 1 in, 1 out]
    }
    n29 = for {
      N: 15 -> [_]
      tunnel: w73 -> [w147]
      tunnel: [w145] -> w69 mode=indexing
      tunnel: 20 ("Numeric") -> [w149]
      tunnel: [w143] -> w25
      tunnel: [w141] -> _ mode=indexing
      tunnel: w26 -> [w140]
      i -> [w151]
      w141 = 4 ("length (rest)")
      n30 = Multiply(x=w141, y=w151) -> (x*y=w148:i32)
      n31 = Add(x=w149, y=w148) -> (x+y=w150:i32)
      n32 = String Subset(string=w147, offset (0)=w150, length (rest)=w141) -> (substring=w146:string)
      n33 = Unflatten From String(type=sgl 0.0, binary string=w146, byte order (0:big-endian, network order)=T1."native, host order" ("byte order (0:big-endian, network order) 2"), error in (no error)=w140) -> (value=w145:sgl, error out=w143:errorcluster)  [unwired: 1 in, 1 out]
    }
    n34 = for {
      N: 15 -> [_]
      tunnel: w73 -> [w125]
      tunnel: [w121] -> w68 mode=indexing
      tunnel: 80 ("Numeric") -> [w127]
      tunnel: [w120] -> w24
      tunnel: w25 -> [w119]
      i -> [w130]
      w128 = 4 ("length (rest)")
      n35 = Multiply(x=w128, y=w130) -> (x*y=w126:i32)
      n36 = Add(x=w127, y=w126) -> (x+y=w129:i32)
      n37 = String Subset(string=w125, offset (0)=w129, length (rest)=w128) -> (substring=w122:string)
      n38 = Unflatten From String(type=sgl 0.0, binary string=w122, byte order (0:big-endian, network order)=T1."native, host order" ("byte order (0:big-endian, network order) 2"), error in (no error)=w119) -> (value=w121:sgl, error out=w120:errorcluster)  [unwired: 1 in, 1 out]
    }
    n39 = for {
      N: 3 -> [_]
      tunnel: w73 -> [w102]
      tunnel: [w101] -> w67 mode=indexing
      tunnel: [w100] -> _
      tunnel: 140 ("Numeric") -> [w95]
      tunnel: w24 -> [w94]
      i -> [w105]
      w96 = 2 ("length (rest)")
      n40 = Multiply(x=w96, y=w105) -> (x*y=w103:i32)
      n41 = Add(x=w95, y=w103) -> (x+y=w104:i32)
      n42 = String Subset(string=w102, offset (0)=w104, length (rest)=w96) -> (substring=w98:string)
      n43 = Unflatten From String(type=u16 0, binary string=w98, byte order (0:big-endian, network order)=T1."native, host order" ("byte order (0:big-endian, network order) 2"), error in (no error)=w94) -> (value=w101:u16, error out=w100:errorcluster)  [unwired: 1 in, 1 out]
    }
    n44 = Interleave 1D Arrays(w69, w68) -> (w64:sgl[])
    n45 = Index Array(array=w67) -> (element #1=w56:u16, element #2=w55:u16, element #3=w57:u16)  [unwired: 3 in]
    n46 = Build Array (concatenate)(w65, w64, w48, w47, w60, w57, w56, w55) -> (w66:sgl[])
    n47 = Format Into String(format string=w46, w65) -> (resulting string=w54:string)  [unwired: 2 in, 1 out]
    n48 = Array To Spreadsheet String(array=w64, 3:"%8.2f" ("format string")) -> (spreadsheet string=w36:string)  [unwired: 1 in]
    n49 = Format Into String(format string=w46, w48) -> (resulting string=w45:string)  [unwired: 2 in, 1 out]
    n50 = Array To Spreadsheet String(array=w47, 3:w46) -> (spreadsheet string=w44:string)  [unwired: 1 in]
    n51 = Format Into String(format string="%04x" ("initial string"), initial string="0x", w60) -> (resulting string=w53:string)  [unwired: 1 in, 1 out]
    n52 = Format Into String(format string="%02x" ("initial string"), initial string="0x", w57) -> (resulting string=w52:string)  [unwired: 1 in, 1 out]
    n53 = Format Into String(w56) -> (resulting string=w51:string)  [unwired: 3 in, 1 out]
    n54 = Format Into String(w55) -> (resulting string=w50:string)  [unwired: 3 in, 1 out]
    n55 = Reverse String(1:w36) -> (0:w37:string)
    n56 = Reverse String(1:w44) -> (0:w43:string)
    n57 = String Subset(string=w37, offset (0)=2) -> (substring=w39:string)  [unwired: 1 in]
    n58 = String Subset(string=w43, offset (0)=2) -> (substring=w41:string)  [unwired: 1 in]
    n59 = Reverse String(1:w39) -> (0:w35:string)
    n60 = Reverse String(1:w41) -> (0:w40:string)
    n61 = Greater Than 0?(x=w31) -> (x > 0?=w32:bool)
    n62 = Concatenate Strings(w54, w33, w35, w33, w45, w33, w40, w33, w53, w33, w52, w33, w51, w33, w50, "\r\n") -> (w49:string)
  }
  "reserved" <- w22
  "count" <- w16
  "max_min" <- w21
  "cycles" <- w20
  "size_status" <- w19
  "cycle period" <- w18
  "M" <- w15
  "Ph" <- w17
  "to_logfile" <- w14
  "to logfile" <- w13
  n63 = Array Size(array=w2) -> (size(s)=w12:i32)
  n64 = Less?(x=w12, y=3) -> (x < y?=w10:bool)
  n65 = feedback #2() -> (w9:u16[])  [unwired: 1 in]
  n66 = Select(t=w9, s=w10, f=w2) -> (s? t:f=w1:u16[])
  "status" <- w1
  n67 = feedback-in #2(w1) -> ()
